vi "AppendReadWaveforms.vi"(10 "WFM in":waveform(dbl)[](array[waveform]), 11 "index of element":i32) -> (2 "WFM out":waveform(dbl)[](array[waveform]), 3 "x = y?":bool)   [LabVIEW 2019, in "DAQ_Manager.lvclass"]
uses:
  DAQ_Manager.lvclass
  DAQ/Typedefs/PublicEvents--DAQ.Read.ctl
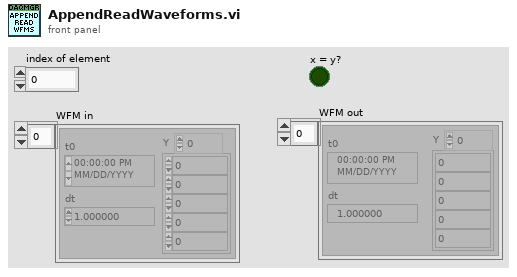
[diagram p1: front panel]
types:
  T1 = typedef "DAQ.lvclass/PublicEvents--DAQ.Read.ctl" = waveform(dbl)[]
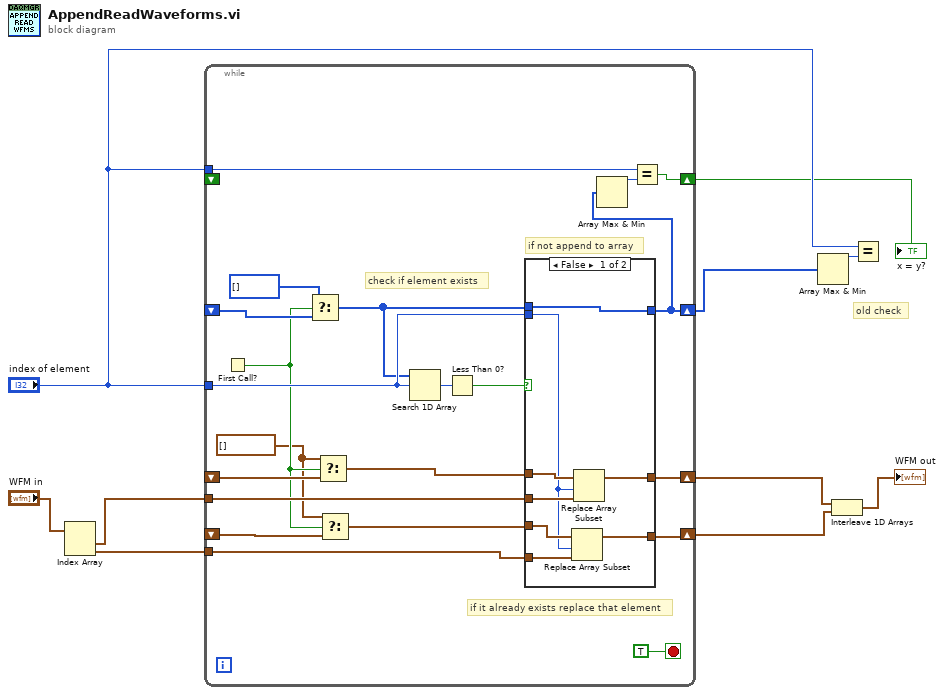
[diagram p0: block diagram]
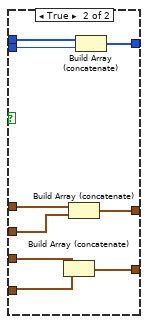
[diagram p2: hidden frame]
diagram:
  # "old check"
  n1 = Index Array(array="WFM in") -> (element #1=w5:waveform(dbl), element #2=w4:waveform(dbl))  [unwired: 2 in]
  n2 = while {
    tunnel: w5 -> [w21]
    tunnel: "index of element" -> [w30]
    shift-right: [w19] -> w10
    shift-left: _ -> [w23]
    shift-right: [w28] -> w3
    shift-left: _ -> [w25]
    tunnel: "index of element" -> [w18]
    shift-right: [w17] -> w7
    shift-left: _ -> [_]
    shift-right: [w11] -> w2
    shift-left: _ -> [w13]
    tunnel: w4 -> [w16]
    stop <- TRUE stop-if-true
    w14 = T1 [] ("t")
    # "if not append to array"
    # "check if element exists"
    # "if it already exists replace that element"
    n3 = First Call?() -> (First Call?: T/F=w15:bool)
    n4 = Select(t=i32[] [], s=w15, f=w23) -> (s? t:f=w22:i32[])
    n5 = Select(t=w14, s=w15, f=w25) -> (s? t:f=w24:T1)
    n6 = Select(t=w14, s=w15, f=w13) -> (s? t:f=w12:T1)
    n7 = Search 1D Array(1D array=w22, element=w30) -> (index of element=w29:i32)  [unwired: 1 in]
    n8 = Less Than 0?(x=w29) -> (x < 0?=w27:bool)
    n9 = case shown="False" w27 {
      tunnel: [w37 w48] -> w19
      tunnel: w30 -> [w32 w47]
      tunnel: w22 -> [w37 w46]
      tunnel: w21 -> [w39 w45]
      tunnel: [w38 w44] -> w28
      tunnel: w24 -> [w36 w43]
      tunnel: w16 -> [w35 w41]
      tunnel: w12 -> [w34 w42]
      tunnel: [w33 w40] -> w11
      frame False {
        n10 = Replace Array Subset(array=w34, new element=w35, index=w32) -> (w33:T1)
        n11 = Replace Array Subset(array=w36, new element=w39, index=w32) -> (w38:T1)
      }
      frame True {
        n12 = Build Array (concatenate)(w42, w41) -> (w40:T1)
        n13 = Build Array (concatenate)(w43, w45) -> (w44:T1)
        n14 = Build Array (concatenate)(w46, w47) -> (w48:i32[])
      }
    }
    n15 = Array Max & Min(array=w19) -> (max value=w20:i32)  [unwired: 3 out]
    n16 = Equal?(x=w18, y=w20) -> (x = y?=w17:bool)
  }
  "x = y?" <- w7
  n17 = Array Max & Min(array=w10) -> (max value=w9:i32)  [unwired: 3 out]
  n18 = Interleave 1D Arrays(w3, w2) -> (→"WFM out":T1)
  n19 = Equal?(x="index of element", y=w9) -> ()  [unwired: 1 out]
